vi "Send CAN Message.vi"(7 "Number of Retries":i32=5, 8 "error in (no error)":errorcluster, 10 "payload":u8[](array[numeric]), 11 "Peltier In":refnum<class "Peltier.lvclass">) -> (0 "error out":errorcluster, 2 "Reply":T1[](array[typedef]) {"payload" format="%x"; "timestamp" format="%<%.7X\n%x>T"; "type" items=["CAN Data"=0, "CAN Remote"=1, "CAN Bus Error"=2, "J1939 Data"=192, "Delay"=224, "Log Trigger"=225, "Start Trigger"=226]; "identifier" format="%x"}, 3 "Peltier Out":refnum<class "Peltier.lvclass">)   [LabVIEW 2015, in "Peltier.lvclass"]
doc: "This VI sends a CAN frame to a device through the CAN network and recieves a frame back as a response. This VI is to facilitate the communication ONLY. The custom error handling of every message must be handled in the owning VI"
uses:
  Peltier.lvclass
  <vilib>/xnet/xnet.llb/XNET Frame CAN.ctl
  <vilib>/xnet/xnet.llb/XNET Frame Type CAN.ctl
  Peltier.lvclass/Peltier.ctl
  <vilib>/xnet/xnet.llb/XNET Write (Frame CAN).vi
  <vilib>/xnet/xnet.llb/XNET Read (Frame CAN).vi
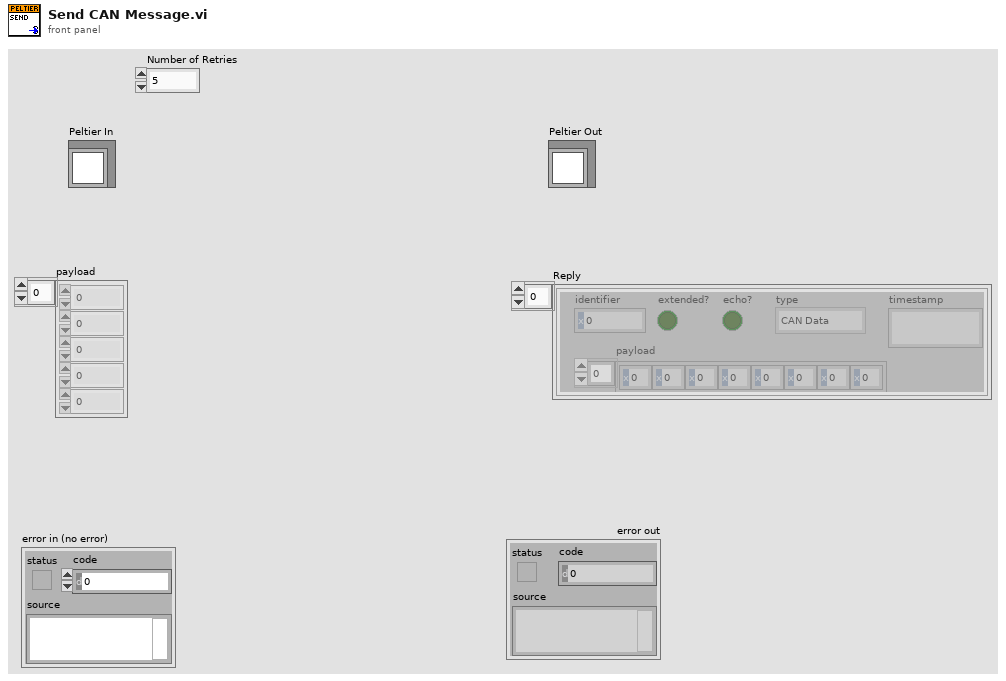
[diagram p1: front panel]
types:
  T1 = typedef "XNET Frame CAN.ctl" = cluster{"timestamp":timestamp, "payload":u8[], "identifier":u32, "type":T2, "extended?":bool, "echo?":bool}
  T2 = typedef "XNET Frame Type CAN.ctl" = u8
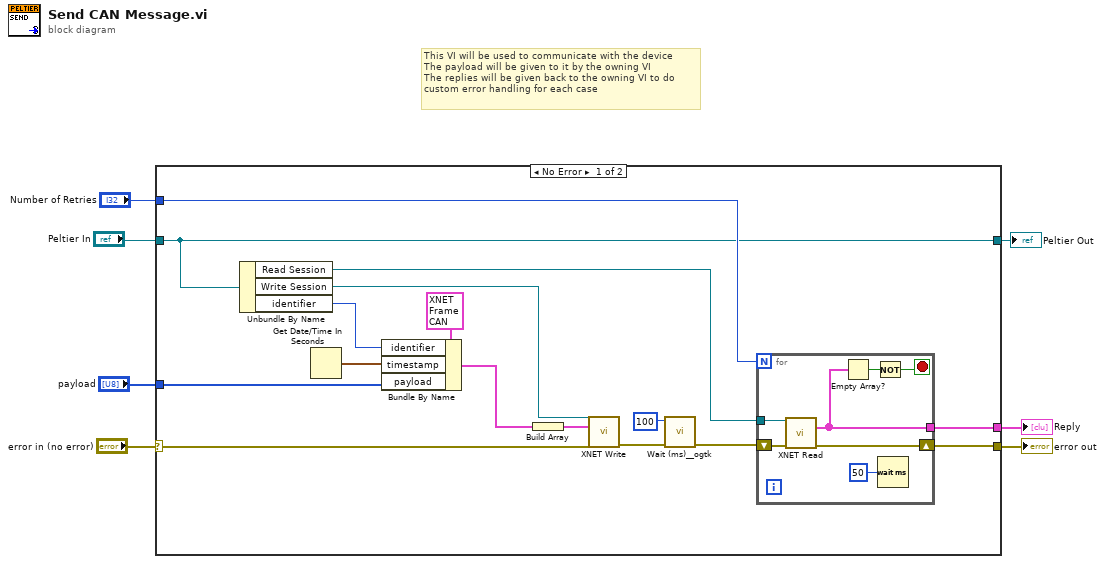
[diagram p0: block diagram]
diagram:
  # "This VI will be used to communicate with the device\nThe payload will be given to it by the owning VI\nThe replies will be given back to the owning VI to do\ncustom error handling for each case"
  n1 = case shown="No Error" "error in (no error)" {
    selector: "error in (no error)" -> [w18 w32]
    tunnel: [w17 w32] -> w7
    tunnel: "Peltier In" -> [w8 w31]
    tunnel: [w8 w31] -> w1
    tunnel: "payload" -> [w13 _]
    tunnel: [w10 _] -> w4
    tunnel: "Number of Retries" -> [w9 _]
    frame No Error {
      n2 = Unbundle By Name(w8) -> ("Read Session"=w20:refnum<k21>, "Write Session"=w23:refnum<k21>, "identifier"=w15:u32)
      n3 = Get Date/Time In Seconds() -> (seconds since 1Jan1904=w14:timestamp)
      n4 = Bundle By Name(cluster=T1 {"timestamp"=timestamp(0 s since 1904-01-01), "payload"=[], "identifier"=0, "type"=0, "extended?"=FALSE, "echo?"=FALSE} ("CAN frame"), "identifier"=w15, "timestamp"=w14, "payload"=w13) -> (w12:T1)
      n5 = Build Array(w12) -> (w11:T1[])
      n6 = call-poly <vilib>:"XNET Write.vi"("session in"=w23, "data"=w11, "error in (no error)"=w18) -> ("error out"=w22:errorcluster)  [unwired: 12 out]
      n7 = call <userlib>:"Wait (ms)__ogtk.vi"("error in (no error)"=w22, "milliseconds to wait"=u32 100) -> ("error out"=w19:errorcluster)  [unwired: 8 in, 1 out]
      n8 = for {
        N: w9 -> [_]
        tunnel: w20 -> [w30]
        shift-right: [w28] -> w17
        shift-left: w19 -> [w29]
        tunnel: [w25] -> w10
        stop <- w26 stop-if-true
        n9 = call-poly <vilib>:"XNET Read.vi"("session in"=w30, "error in (no error)"=w29) -> ("data"=w25:T1[], "error out"=w28:errorcluster)  [unwired: 12 out]
        n10 = Empty Array?(array=w25) -> (empty?=w27:bool)
        n11 = Not(x=w27) -> (.not. x?=w26:bool)
        n12 = Wait (ms)(milliseconds to wait=u32 50) -> ()  [unwired: 1 out]
      }
    }
    frame Error {
    }
  }
  "error out" <- w7
  "Reply" <- w4
  "Peltier Out" <- w1
